vi "Experiment 7.vi"() -> ()   [LabVIEW 2026]
doc: "Experiment 7"
uses:
  <vilib>/Analysis/baseanly.llb/Mean (DBL).vi
  <vilib>/Analysis/NI_AALBase.lvlib
panel:
  out "No. Of Iterations Executed - Loop 4":i32
  out "Output - Loop 4":dbl[](array[numeric]) format="%.3f"
  out "No. Of Iterations Executed - Loop 3":i32
  out "Output - Loop 3":dbl[](array[numeric]) format="%.3f"
  out "Avg. No. Of Iterations Executed - All Loops":dbl format="%.1f"
  out "No. Of Iterations Executed - Loop 2":i32
  out "Output - Loop 2":dbl[](array[numeric]) format="%.3f"
  out "No. Of Iterations Executed - Loop 1":i32
  out "Output - Loop 1":dbl[](array[numeric]) format="%.3f"
  out "Stop VI?":bool
  # "Experiment 7"
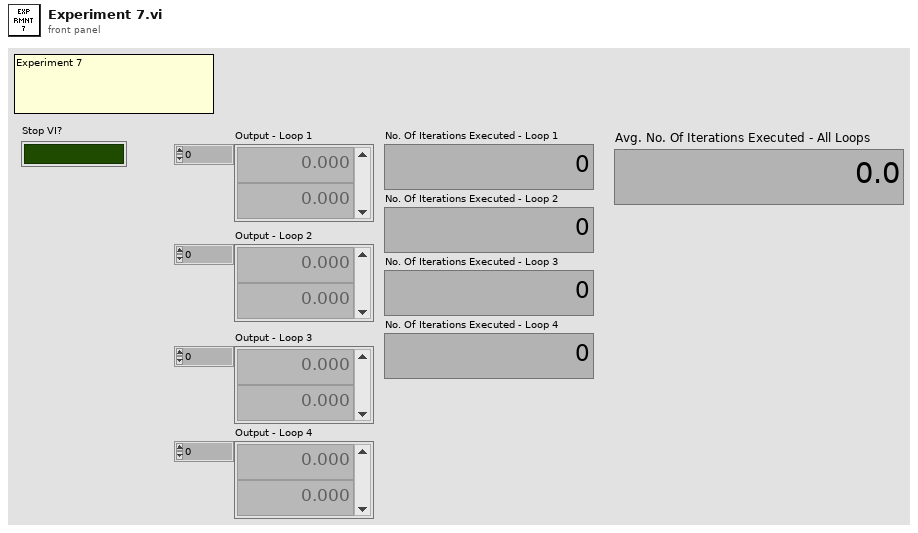
[diagram p1: front panel]
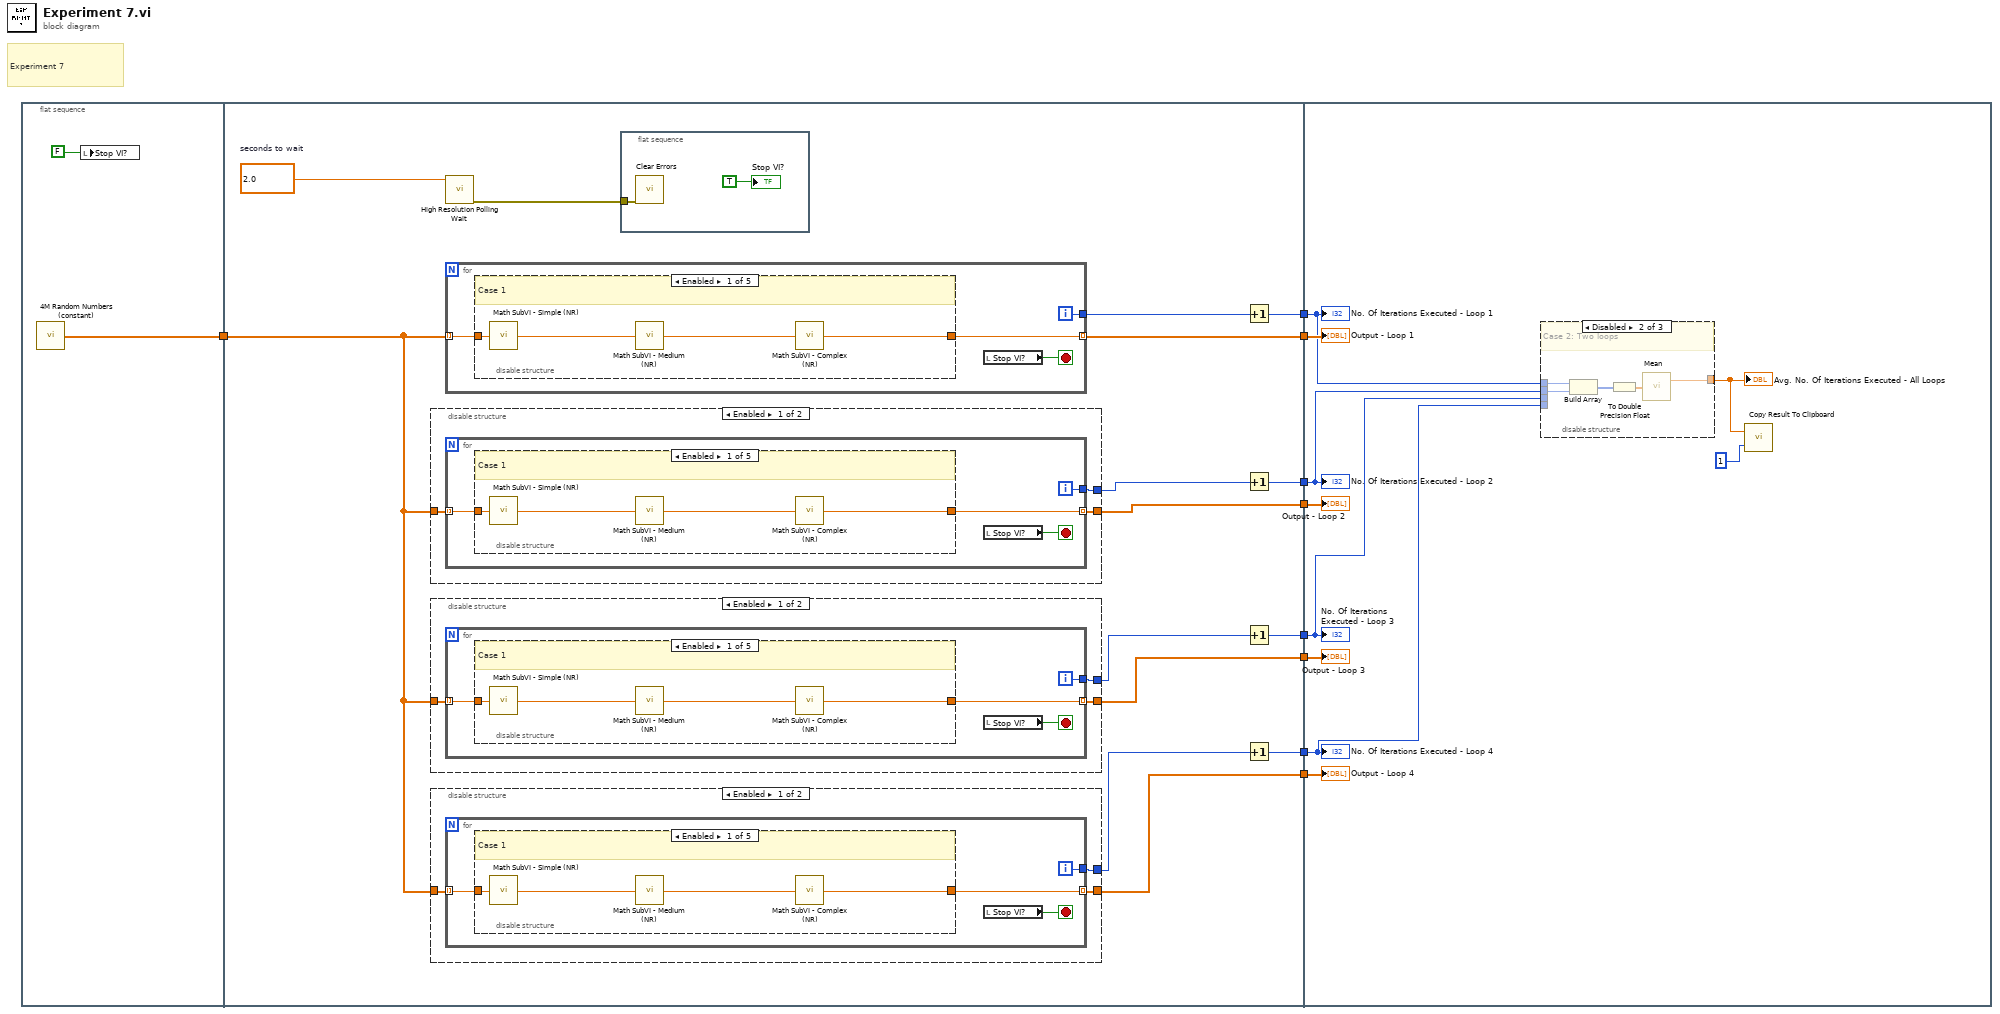
[diagram p0: block diagram]
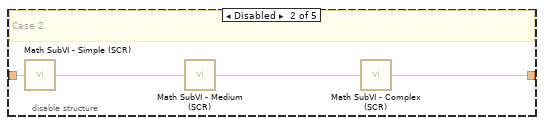
[diagram p2: hidden frame]
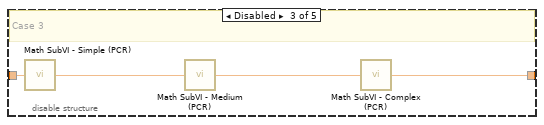
[diagram p3: hidden frame]
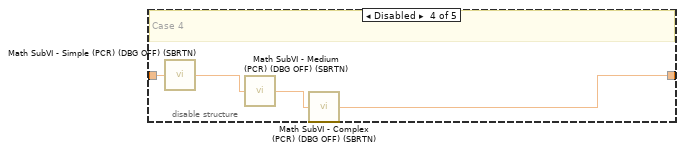
[diagram p4: hidden frame]
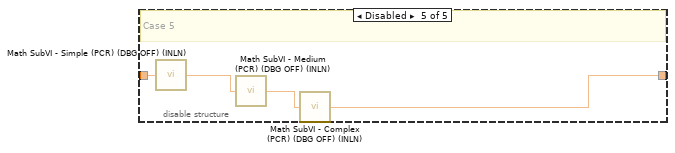
[diagram p5: hidden frame]
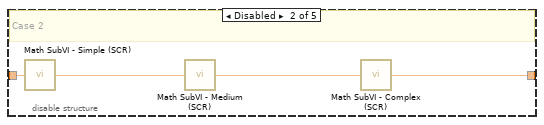
[diagram p7: hidden frame]
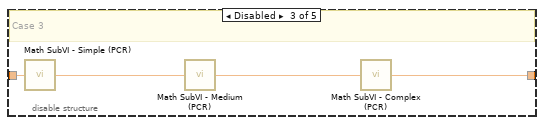
[diagram p8: hidden frame]
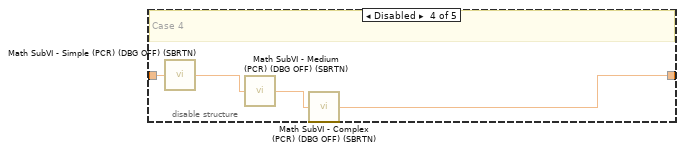
[diagram p9: hidden frame]
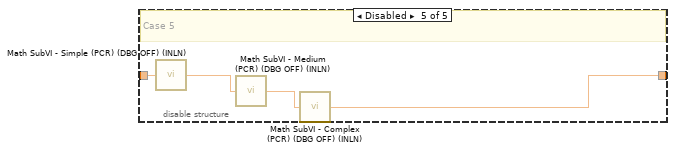
[diagram p10: hidden frame]
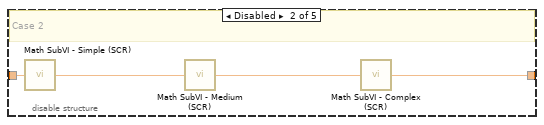
[diagram p12: hidden frame]
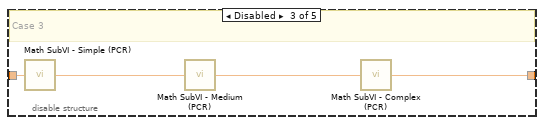
[diagram p13: hidden frame]
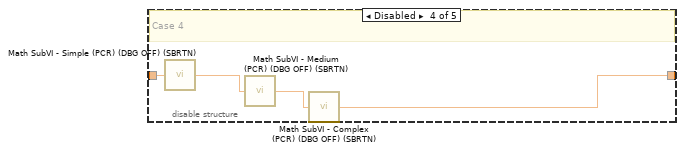
[diagram p14: hidden frame]
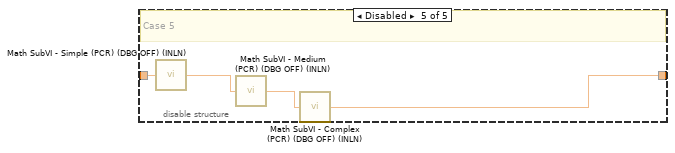
[diagram p15: hidden frame]
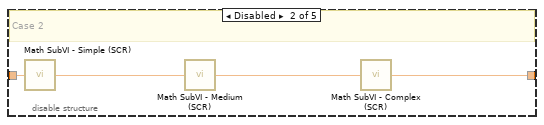
[diagram p17: hidden frame]
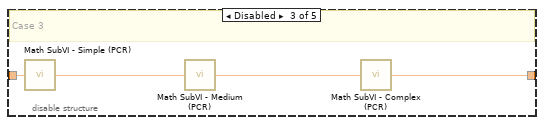
[diagram p18: hidden frame]
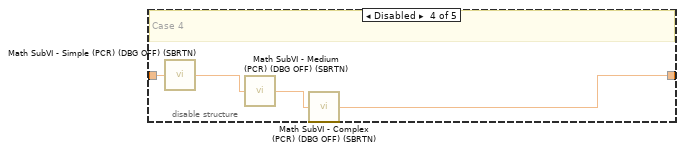
[diagram p19: hidden frame]
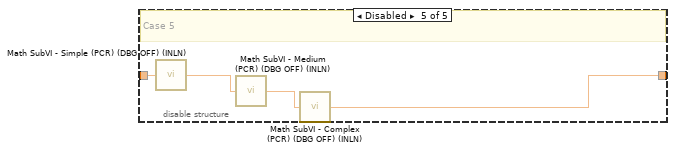
[diagram p20: hidden frame]
diagram:
  # "Experiment 7"
  n1 = flat-sequence {
    tunnel: [w10] -> w1
    tunnel: [w24] -> w9
    tunnel: [w22] -> w8
    tunnel: [w21] -> w7
    tunnel: [w17] -> w6
    tunnel: [w20] -> w5
    tunnel: [w15] -> w4
    tunnel: [w13] -> w3
    tunnel: [w19] -> w2
    tunnel: w1 -> [w12]
    tunnel: w9 -> [w143]
    tunnel: w8 -> [w141]
    tunnel: w7 -> [w140]
    tunnel: w6 -> [w142]
    tunnel: w5 -> [w135]
    tunnel: w4 -> [w138]
    tunnel: w3 -> [w137]
    tunnel: w2 -> [w134]
    frame #0 {
      n2 = call "4M Random Numbers (constant).vi"() -> ("4M Random Numbers"=w10:dbl[])
      n3 = local write "Stop VI?"(FALSE) -> ()
    }
    frame #1 {
      w26 = 2.0  # seconds to wait
      n4 = disable-structure shown="Enabled" {
        disable-tunnel: [w83 _] -> w18
        disable-tunnel: [w82 _] -> w17
        disable-tunnel: w12 -> [w81 _]
        frame Enabled {
          n5 = for {
            tunnel: w81 -> [w85] mode=indexing
            tunnel: [w84] -> w82 mode=indexing
            tunnel: [w86] -> w83
            i -> [w86]
            stop <- w87 stop-if-true
            n6 = disable-structure shown="Enabled" {
              disable-tunnel: w85 -> [w91 w95 w99 w103 w107]
              disable-tunnel: [w88 w92 w96 w100 w104] -> w84
              frame Enabled {
                # "Case 1"
                n7 = call "Math SubVI - Simple (NR).vi"("Input"=w91) -> ("Output"=w89:dbl)
                n8 = call "Math SubVI - Medium (NR).vi"("Input"=w89) -> ("Output"=w90:dbl)
                n9 = call "Math SubVI - Complex (NR).vi"("Input"=w90) -> ("Output"=w88:dbl)
              }
              frame Disabled {
                # "Case 2"
                n10 = call "Math SubVI - Simple (SCR).vi"("Input"=w95) -> ("Output"=w93:dbl)
                n11 = call "Math SubVI - Medium (SCR).vi"("Input"=w93) -> ("Output"=w94:dbl)
                n12 = call "Math SubVI - Complex (SCR).vi"("Input"=w94) -> ("Output"=w92:dbl)
              }
              frame Disabled {
                # "Case 3"
                n13 = call "Math SubVI - Simple (PCR).vi"("Input"=w99) -> ("Output"=w97:dbl)
                n14 = call "Math SubVI - Medium (PCR).vi"("Input"=w97) -> ("Output"=w98:dbl)
                n15 = call "Math SubVI - Complex (PCR).vi"("Input"=w98) -> ("Output"=w96:dbl)
              }
              frame Disabled {
                # "Case 4"
                n16 = call "Math SubVI - Simple (PCR) (DBG OFF) (SBRTN).vi"("Input"=w103) -> ("Output"=w101:dbl)
                n17 = call "Math SubVI - Medium (PCR) (DBG OFF) (SBRTN).vi"("Input"=w101) -> ("Output"=w102:dbl)
                n18 = call "Math SubVI - Complex (PCR) (DBG OFF) (SBRTN).vi"("Input"=w102) -> ("Output"=w100:dbl)
              }
              frame Disabled {
                # "Case 5"
                n19 = call "Math SubVI - Simple (PCR) (DBG OFF) (INLN).vi"("Input"=w107) -> ("Output"=w105:dbl)
                n20 = call "Math SubVI - Medium (PCR) (DBG OFF) (INLN).vi"("Input"=w105) -> ("Output"=w106:dbl)
                n21 = call "Math SubVI - Complex (PCR) (DBG OFF) (INLN).vi"("Input"=w106) -> ("Output"=w104:dbl)
              }
            }
            n22 = local read "Stop VI?"() -> (w87:bool)
          }
        }
        frame Disabled {
        }
      }
      n23 = disable-structure shown="Enabled" {
        disable-tunnel: [w56 _] -> w16
        disable-tunnel: [w55 _] -> w15
        disable-tunnel: w12 -> [w54 _]
        frame Enabled {
          n24 = for {
            tunnel: w54 -> [w58] mode=indexing
            tunnel: [w57] -> w55 mode=indexing
            tunnel: [w59] -> w56
            i -> [w59]
            stop <- w60 stop-if-true
            n25 = disable-structure shown="Enabled" {
              disable-tunnel: w58 -> [w64 w68 w72 w76 w80]
              disable-tunnel: [w61 w65 w69 w73 w77] -> w57
              frame Enabled {
                # "Case 1"
                n26 = call "Math SubVI - Simple (NR).vi"("Input"=w64) -> ("Output"=w62:dbl)
                n27 = call "Math SubVI - Medium (NR).vi"("Input"=w62) -> ("Output"=w63:dbl)
                n28 = call "Math SubVI - Complex (NR).vi"("Input"=w63) -> ("Output"=w61:dbl)
              }
              frame Disabled {
                # "Case 2"
                n29 = call "Math SubVI - Simple (SCR).vi"("Input"=w68) -> ("Output"=w66:dbl)
                n30 = call "Math SubVI - Medium (SCR).vi"("Input"=w66) -> ("Output"=w67:dbl)
                n31 = call "Math SubVI - Complex (SCR).vi"("Input"=w67) -> ("Output"=w65:dbl)
              }
              frame Disabled {
                # "Case 3"
                n32 = call "Math SubVI - Simple (PCR).vi"("Input"=w72) -> ("Output"=w70:dbl)
                n33 = call "Math SubVI - Medium (PCR).vi"("Input"=w70) -> ("Output"=w71:dbl)
                n34 = call "Math SubVI - Complex (PCR).vi"("Input"=w71) -> ("Output"=w69:dbl)
              }
              frame Disabled {
                # "Case 4"
                n35 = call "Math SubVI - Simple (PCR) (DBG OFF) (SBRTN).vi"("Input"=w76) -> ("Output"=w74:dbl)
                n36 = call "Math SubVI - Medium (PCR) (DBG OFF) (SBRTN).vi"("Input"=w74) -> ("Output"=w75:dbl)
                n37 = call "Math SubVI - Complex (PCR) (DBG OFF) (SBRTN).vi"("Input"=w75) -> ("Output"=w73:dbl)
              }
              frame Disabled {
                # "Case 5"
                n38 = call "Math SubVI - Simple (PCR) (DBG OFF) (INLN).vi"("Input"=w80) -> ("Output"=w78:dbl)
                n39 = call "Math SubVI - Medium (PCR) (DBG OFF) (INLN).vi"("Input"=w78) -> ("Output"=w79:dbl)
                n40 = call "Math SubVI - Complex (PCR) (DBG OFF) (INLN).vi"("Input"=w79) -> ("Output"=w77:dbl)
              }
            }
            n41 = local read "Stop VI?"() -> (w60:bool)
          }
        }
        frame Disabled {
        }
      }
      n42 = disable-structure shown="Enabled" {
        disable-tunnel: [w29 _] -> w14
        disable-tunnel: [w28 _] -> w13
        disable-tunnel: w12 -> [w27 _]
        frame Enabled {
          n43 = for {
            tunnel: w27 -> [w31] mode=indexing
            tunnel: [w30] -> w28 mode=indexing
            tunnel: [w32] -> w29
            i -> [w32]
            stop <- w33 stop-if-true
            n44 = disable-structure shown="Enabled" {
              disable-tunnel: w31 -> [w37 w41 w45 w49 w53]
              disable-tunnel: [w34 w38 w42 w46 w50] -> w30
              frame Enabled {
                # "Case 1"
                n45 = call "Math SubVI - Simple (NR).vi"("Input"=w37) -> ("Output"=w35:dbl)
                n46 = call "Math SubVI - Medium (NR).vi"("Input"=w35) -> ("Output"=w36:dbl)
                n47 = call "Math SubVI - Complex (NR).vi"("Input"=w36) -> ("Output"=w34:dbl)
              }
              frame Disabled {
                # "Case 2"
                n48 = call "Math SubVI - Simple (SCR).vi"("Input"=w41) -> ("Output"=w39:dbl)
                n49 = call "Math SubVI - Medium (SCR).vi"("Input"=w39) -> ("Output"=w40:dbl)
                n50 = call "Math SubVI - Complex (SCR).vi"("Input"=w40) -> ("Output"=w38:dbl)
              }
              frame Disabled {
                # "Case 3"
                n51 = call "Math SubVI - Simple (PCR).vi"("Input"=w45) -> ("Output"=w43:dbl)
                n52 = call "Math SubVI - Medium (PCR).vi"("Input"=w43) -> ("Output"=w44:dbl)
                n53 = call "Math SubVI - Complex (PCR).vi"("Input"=w44) -> ("Output"=w42:dbl)
              }
              frame Disabled {
                # "Case 4"
                n54 = call "Math SubVI - Simple (PCR) (DBG OFF) (SBRTN).vi"("Input"=w49) -> ("Output"=w47:dbl)
                n55 = call "Math SubVI - Medium (PCR) (DBG OFF) (SBRTN).vi"("Input"=w47) -> ("Output"=w48:dbl)
                n56 = call "Math SubVI - Complex (PCR) (DBG OFF) (SBRTN).vi"("Input"=w48) -> ("Output"=w46:dbl)
              }
              frame Disabled {
                # "Case 5"
                n57 = call "Math SubVI - Simple (PCR) (DBG OFF) (INLN).vi"("Input"=w53) -> ("Output"=w51:dbl)
                n58 = call "Math SubVI - Medium (PCR) (DBG OFF) (INLN).vi"("Input"=w51) -> ("Output"=w52:dbl)
                n59 = call "Math SubVI - Complex (PCR) (DBG OFF) (INLN).vi"("Input"=w52) -> ("Output"=w50:dbl)
              }
            }
            n60 = local read "Stop VI?"() -> (w33:bool)
          }
        }
        frame Disabled {
        }
      }
      n61 = call <vilib>:"High Resolution Polling Wait.vi"("seconds to wait"=w26) -> ("error out"=w25:errorcluster)  [unwired: 10 in]
      n62 = for {
        tunnel: w12 -> [w111] mode=indexing
        tunnel: [w108] -> w24 mode=indexing
        tunnel: [w109] -> w23
        i -> [w109]
        stop <- w110 stop-if-true
        n63 = disable-structure shown="Enabled" {
          disable-tunnel: w111 -> [w115 w119 w123 w127 w131]
          disable-tunnel: [w112 w116 w120 w124 w128] -> w108
          frame Enabled {
            # "Case 1"
            n64 = call "Math SubVI - Simple (NR).vi"("Input"=w115) -> ("Output"=w113:dbl)
            n65 = call "Math SubVI - Medium (NR).vi"("Input"=w113) -> ("Output"=w114:dbl)
            n66 = call "Math SubVI - Complex (NR).vi"("Input"=w114) -> ("Output"=w112:dbl)
          }
          frame Disabled {
            # "Case 2"
            n67 = call "Math SubVI - Simple (SCR).vi"("Input"=w119) -> ("Output"=w117:dbl)
            n68 = call "Math SubVI - Medium (SCR).vi"("Input"=w117) -> ("Output"=w118:dbl)
            n69 = call "Math SubVI - Complex (SCR).vi"("Input"=w118) -> ("Output"=w116:dbl)
          }
          frame Disabled {
            # "Case 3"
            n70 = call "Math SubVI - Simple (PCR).vi"("Input"=w123) -> ("Output"=w121:dbl)
            n71 = call "Math SubVI - Medium (PCR).vi"("Input"=w121) -> ("Output"=w122:dbl)
            n72 = call "Math SubVI - Complex (PCR).vi"("Input"=w122) -> ("Output"=w120:dbl)
          }
          frame Disabled {
            # "Case 4"
            n73 = call "Math SubVI - Simple (PCR) (DBG OFF) (SBRTN).vi"("Input"=w127) -> ("Output"=w125:dbl)
            n74 = call "Math SubVI - Medium (PCR) (DBG OFF) (SBRTN).vi"("Input"=w125) -> ("Output"=w126:dbl)
            n75 = call "Math SubVI - Complex (PCR) (DBG OFF) (SBRTN).vi"("Input"=w126) -> ("Output"=w124:dbl)
          }
          frame Disabled {
            # "Case 5"
            n76 = call "Math SubVI - Simple (PCR) (DBG OFF) (INLN).vi"("Input"=w131) -> ("Output"=w129:dbl)
            n77 = call "Math SubVI - Medium (PCR) (DBG OFF) (INLN).vi"("Input"=w129) -> ("Output"=w130:dbl)
            n78 = call "Math SubVI - Complex (PCR) (DBG OFF) (INLN).vi"("Input"=w130) -> ("Output"=w128:dbl)
          }
        }
        n79 = local read "Stop VI?"() -> (w110:bool)
      }
      n80 = flat-sequence {
        tunnel: w25 -> [w132]
        frame #0 {
          n81 = call <vilib>:"Clear Errors.vi"("error in (no error)"=w132) -> ()  [unwired: 5 in, 2 out]
          "Stop VI?" <- TRUE
        }
      }
      n82 = Increment(x=w23) -> (x+1=w22:i32)
      n83 = Increment(x=w18) -> (x+1=w21:i32)
      n84 = Increment(x=w16) -> (x+1=w20:i32)
      n85 = Increment(x=w14) -> (x+1=w19:i32)
    }
    frame #2 {
      n86 = disable-structure shown="Disabled" {
        disable-tunnel: w141 -> [w145 w150 w157]
        disable-tunnel: w140 -> [_ w149 w156]
        disable-tunnel: [w144 w146 w153] -> w139
        disable-tunnel: w135 -> [_ _ w152]
        disable-tunnel: w134 -> [_ _ w151]
        frame Disabled {
          # "Case 1: One loop"
          n87 = To Double Precision Float(number=w145) -> (double precision float=w144:dbl)
        }
        frame Disabled {
          # "Case 2: Two loops"
          n88 = Build Array(w150, w149) -> (w148:i32[])
          n89 = To Double Precision Float(number=w148) -> (double precision float=w147:dbl[])
          n90 = call-poly <vilib>:"Mean.vi"("X"=w147) -> ("mean"=w146:dbl)  [unwired: 1 out]
        }
        frame Enabled {
          # "Case 3: Four loops"
          n91 = Build Array(w157, w156, w152, w151) -> (w155:i32[])
          n92 = To Double Precision Float(number=w155) -> (double precision float=w154:dbl[])
          n93 = call-poly <vilib>:"Mean.vi"("X"=w154) -> ("mean"=w153:dbl)  [unwired: 1 out]
        }
      }
      "Avg. No. Of Iterations Executed - All Loops" <- w139
      n94 = call "Copy Result To Clipboard.vi"("No. Of Decimal Places (6)"=u32 1, "Input"=w139) -> ()
      "No. Of Iterations Executed - Loop 1" <- w141
      "Output - Loop 1" <- w143
      "No. Of Iterations Executed - Loop 2" <- w140
      "Output - Loop 2" <- w142
      "No. Of Iterations Executed - Loop 3" <- w135
      "Output - Loop 3" <- w138
      "No. Of Iterations Executed - Loop 4" <- w134
      "Output - Loop 4" <- w137
    }
  }
